vi "CPU_klaus_dorman_test.vi"() -> ()   [LabVIEW 2018]
uses:
  CPU_registers.ctl
  memory/CPU_MEM_RAM.vi
  CPU_Port.vi
  memory/CPU_MEM_RAM_WR.vi
  memory/CPU_MEM_VIC-II.vi
  memory/CPU_MEM_SID_WR.vi
  memory/CPU_MEM_CIA 1.vi
  memory/CPU_MEM_CIA 2.vi
  memory/CPU_MEM_Color_WR.vi
panel:
  out "ticks/s":u32 format="%.2p"
  in  "stop":bool
  out "registers":T1 {"P" format="%08b"; "PC" format="%04x"; "SP" format="%02x"; "Y" format="%02x"; "X" format="%02x"; "A" format="%02x"}
  # "This program executes the Klaus Dormann 6502 functional test.\nThe test is a comprehensive validation suite that covers all official\n6502 instructions, addressing modes, and flag behaviors, ensuring\ncycle-accurate emulation across edge cases.\nIt is widely regarded as one of the most complete functional tests\nfor the 6502 CPU, checking thousands of instruction sequences.\nReference: Klaus Dormann's 6502 functional test repository\nhttps://github.com/Klaus2m5/6502_65C02_functional_tests"
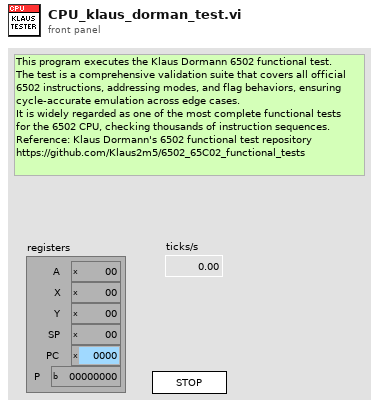
[diagram p1: front panel]
types:
  T1 = typedef "CPU_registers.ctl" = cluster{"A":u8, "X":u8, "Y":u8, "SP":u8, "PC":u16, "P":u8}
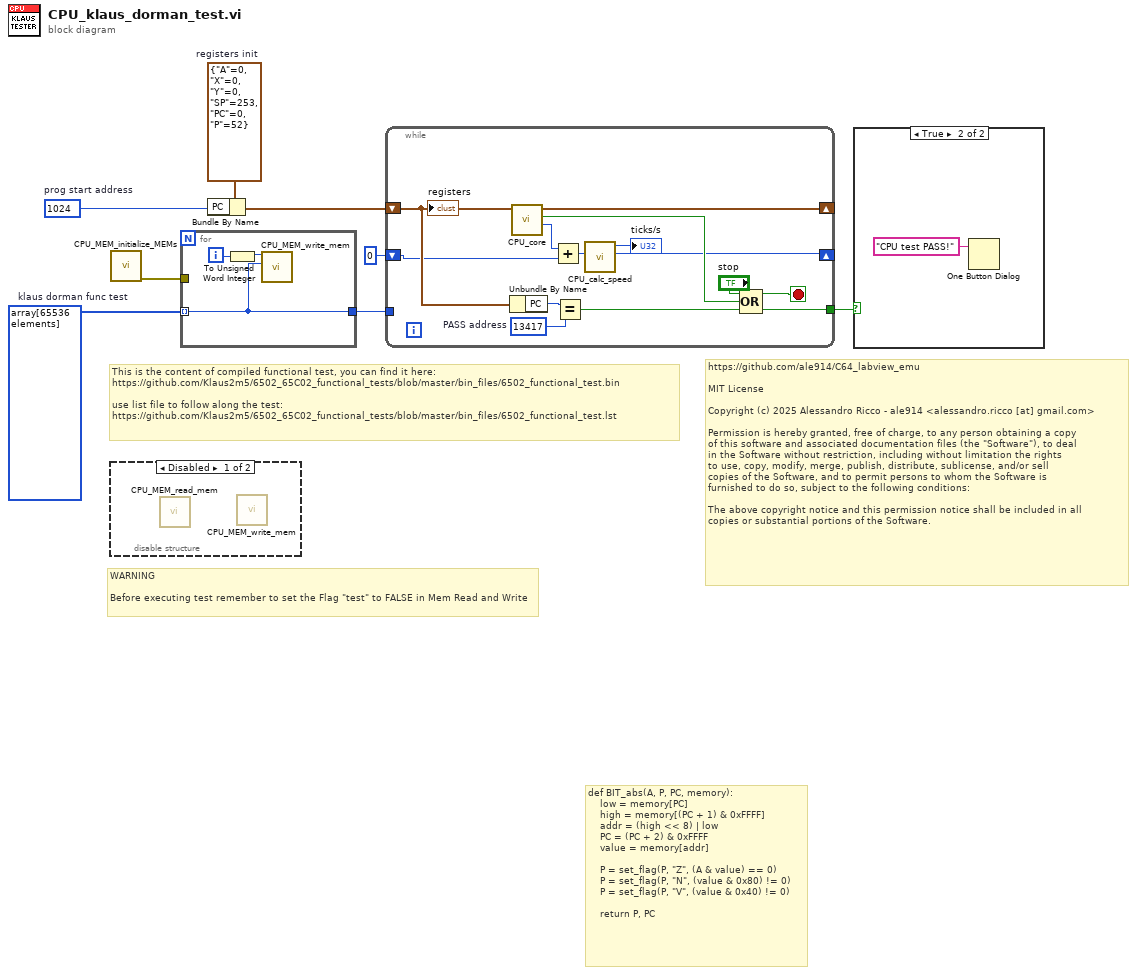
[diagram p0: block diagram]
diagram:
  w7 = u16 1024  # prog start address
  w5 = T1 {"A"=0, "X"=0, "Y"=0, "SP"=253, "PC"=0, "P"=52}  # registers init
  w8 = u8[] array[65536 elements]  # klaus dorman func test
  # "WARNING\n\nBefore executing test remember to set the Flag \"test\" to FALSE in Mem Read and Write"
  # "https://github.com/ale914/C64_labview_emu\n\nMIT License\n\nCopyright (c) 2025 Alessandro Ricco - ale914 <alessandro.ricco [at] gmail.com>\n\nPermission is hereby granted, free of charge, to any person obtaining a copy\nof this software and associated documentation files (the \"Software\"), to deal\nin the Software without restriction, including without limitation the rights\nto use, copy, modify, merge, publish, distribute, sublicense, and/or sell\ncopies of the Software, and to permit persons to whom the Software is\nfurnished to do so, subject to the following conditions:\n\nThe above copyright notice and this permission notice shall be included in all\ncopies or substantial portions of the Software."
  # "This is the content of compiled functional test, you can find it here:\nhttps://github.com/Klaus2m5/6502_65C02_functional_tests/blob/master/bin_files/6502_functional_test.bin\n\nuse list file to follow along the test:\nhttps://github.com/Klaus2m5/6502_65C02_functional_tests/blob/master/bin_files/6502_functional_test.lst"
  # "def BIT_abs(A, P, PC, memory):\n    low = memory[PC]\n    high = memory[(PC + 1) & 0xFFFF]\n    addr = (high << 8) | low\n    PC = (PC + 2) & 0xFFFF\n    value = memory[addr]\n\n    P = set_flag(P, \"Z\", (A & value) == 0)\n    P = set_flag(P, \"N\", (value & 0x80) != 0)\n    P = set_flag(P, \"V\", (value & 0x40) != 0)\n\n    return P, PC"
  n1 = call "CPU_MEM_initialize_MEMs.vi"() -> ("error out"=w6:errorcluster)  [unwired: 11 in]
  n2 = disable-structure shown="Disabled" {
    frame Disabled {
      n3 = call "CPU_MEM_read_mem.vi"() -> ()  [unwired: 11 in, 1 out]
      n4 = call "CPU_MEM_write_mem.vi"() -> ()  [unwired: 12 in]
    }
    frame Enabled {
    }
  }
  n5 = for {
    tunnel: w8 -> [w9] mode=indexing
    tunnel: w6 -> [_]
    tunnel: [w9] -> w3
    i -> [w11]
    n6 = To Unsigned Word Integer(number=w11) -> (unsigned 16bit integer=w10:u16)
    n7 = call "CPU_MEM_write_mem.vi"("value"=w9, "address"=w10) -> ()  [unwired: 10 in]
  }
  n8 = Bundle By Name(cluster=w5, "PC"=w7) -> (w4:T1)
  n9 = while {
    shift-right: [w21] -> _
    shift-left: w4 -> [w19]
    tunnel: w3 -> [_]
    tunnel: [w16] -> w2
    shift-right: [w12] -> _
    shift-left: u32 0 ("clock ticks out") -> [w15]
    stop <- w23 stop-if-true
    w17 = u16 13417  # PASS address
    n10 = Unbundle By Name(w19) -> ("PC"=w18:u16)
    n11 = call "CPU_core.vi"("registers"=w19) -> ("clock ticks"=w14:u8, "error"=w20:bool, "registers"=w21:T1)  [unwired: 8 in]
    n12 = Add(x=w14, y=w15) -> (x+y=w13:u32)
    n13 = Equal?(x=w18, y=w17) -> (x = y?=w16:bool)
    n14 = call "CPU_calc_speed.vi"("clock ticks"=w13) -> ("clock ticks out"=w12:u32, "ticks/s"=→"ticks/s":u32)  [unwired: 9 in]
    n15 = Compound Arithmetic op=OR("stop", w20, w16) -> (w23:bool)
    "registers" <- w19
  }
  n16 = case shown="True" w2 {
    frame False {
    }
    frame True {
      n17 = One Button Dialog(message="CPU test PASS!") -> ()  [unwired: 1 in, 1 out]
    }
  }
